vi "Tusk.IsTopLevel.vi"(8 "error in (no error)":errorcluster, 11 "Tusk in":refnum<class "Tusk.lvclass">) -> (0 "error out":errorcluster, 2 "Is Top Level?":bool, 3 "Tusk out":refnum<class "Tusk.lvclass">)   [LabVIEW 2018, in "Application.lvlib" / "Tusk.lvclass"]
uses:
  Tusk.lvclass
  Tusk.lvclass/Tusk.ctl
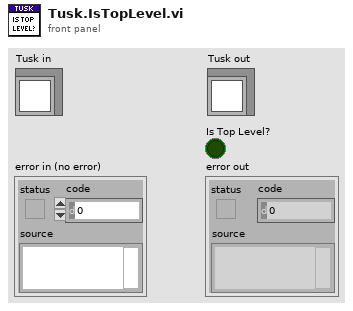
[diagram p1: front panel]
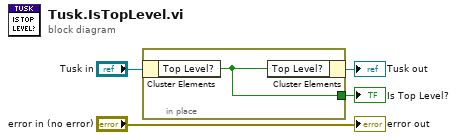
[diagram p0: block diagram]
diagram:
  n1 = in-place {
    in-place-border: [w5] -> w1
    n2 = in-place-cluster #1("Tusk in") -> ("Top Level?"=w5:bool)
    n3 = in-place-cluster #1("Top Level?"=w5) -> (→"Tusk out":refnum<class "Tusk.lvclass">)
  }
  "Is Top Level?" <- w1
  "error out" <- "error in (no error)"
